vi "DriveSet_Test_Actions.vi"(8 "Do PID test":bool, 9 "Do Ka  Test":bool, 10 "Do 0.8 output":bool, 11 "Do 0.2 output":bool) -> ()   [LabVIEW 2023]
doc: "set speed demand variable for drive (called in human)"
uses:
  DriveGlobal.vi
  <vilib>/Rock Robotics/WPI/ThirdParty/JAS_Junk/TrajLib/Trajectory_Library.lvlib
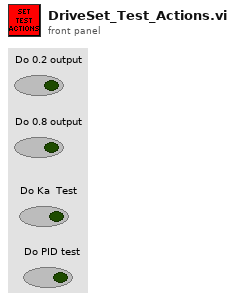
[diagram p1: front panel]
types:
  T1 = typedef "Trajectory_Library.lvlib/CHASSIS_SPEEDS.ctl" = cluster{"vX":dbl, "vY":dbl, "vOmega":dbl}
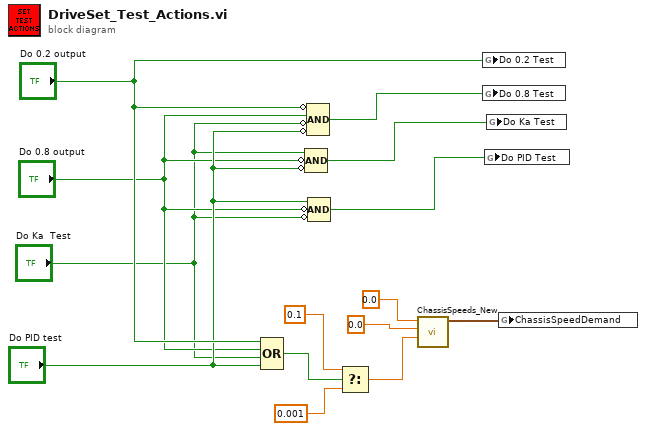
[diagram p0: block diagram]
diagram:
  n1 = Compound Arithmetic op=OR("Do 0.2 output", "Do 0.8 output", "Do Ka  Test", "Do PID test") -> (w9:bool)
  n2 = Compound Arithmetic op=AND("Do Ka  Test", invert "Do 0.8 output", invert "Do PID test") -> (w5:bool)
  n3 = Compound Arithmetic op=AND(invert "Do 0.2 output", "Do 0.8 output", invert "Do Ka  Test", invert "Do PID test") -> (w6:bool)
  n4 = Compound Arithmetic op=AND("Do PID test", invert "Do 0.8 output", invert "Do Ka  Test") -> (w1:bool)
  n5 = Select(t=0.1, s=w9, f=0.001) -> (s? t:f=w11:dbl)
  n6 = call <vilib>:"ChassisSpeeds_New.vi"("vAngular"=w11, "vY"=0.0, "vX"=0.0) -> ("CHASSIS"=w14:T1)  [unwired: 8 in]
  n7 = global write "DriveGlobal.vi" "Do 0.2 Test"("Do 0.2 output") -> ()
  n8 = global write "DriveGlobal.vi" "Do 0.8 Test"(w6) -> ()
  n9 = global write "DriveGlobal.vi" "Do PID Test"(w1) -> ()
  n10 = global write "DriveGlobal.vi" "Do Ka Test"(w5) -> ()
  n11 = global write "DriveGlobal.vi" "ChassisSpeedDemand"(w14) -> ()
